vi "respuesta read adc.vi"(8 "error in (no error)":errorcluster, 11 "NXP in":refnum<class "NXP.lvclass">) -> (0 "error out":errorcluster, 2 "salida":string, 3 "NXP out":refnum<class "NXP.lvclass">)   [LabVIEW 2019, in "NXP.lvclass"]
uses:
  NXP.lvclass
  NXP.lvclass/NXP.ctl
  Serial Device.lvclass
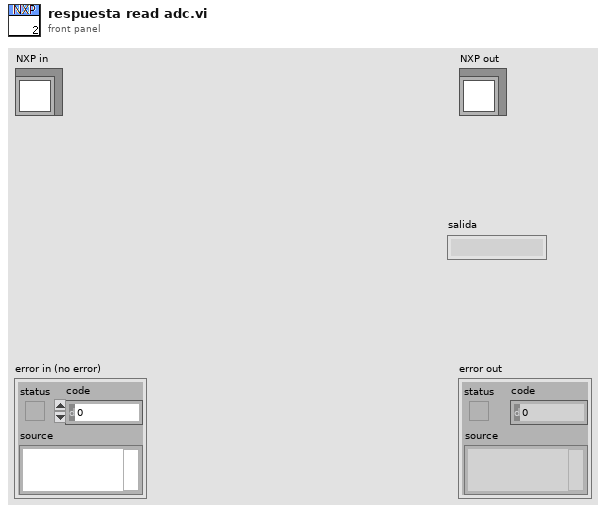
[diagram p1: front panel]
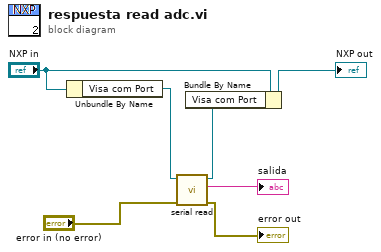
[diagram p0: block diagram]
diagram:
  n1 = Unbundle By Name("NXP in") -> ("Visa com Port"=w7:refnum<visa-resource-name>)
  n2 = call "serial read.vi"("error in (no error)"="error in (no error)", "VISA resource name"=w7) -> ("error out"=→"error out":errorcluster, "respuesta serial"=→"salida":string, "VISA resource nameout"=w5:refnum<visa-resource-name>)  [unwired: 7 in]
  n3 = Bundle By Name(cluster="NXP in", "Visa com Port"=w5) -> (→"NXP out":refnum<class "NXP.lvclass">)
